vi "stable test.vi"() -> ()   [LabVIEW 2016]
uses:
  <vilib>/DAQmx/read.llb/DAQmx Read (Analog Wfm 1Chan NSamp).vi
  <vilib>/DAQmx/miscellaneous.llb/DAQmx Fill In Error Info.vi
  <resource>/objmgr/daqmx.rc
panel:
  out "data 2":waveform(dbl)
  out "Waveform Graph":waveform(dbl)(graph)
  out "data":dbl[](array[numeric]) format="%0.2f"
  out "error out":errorcluster
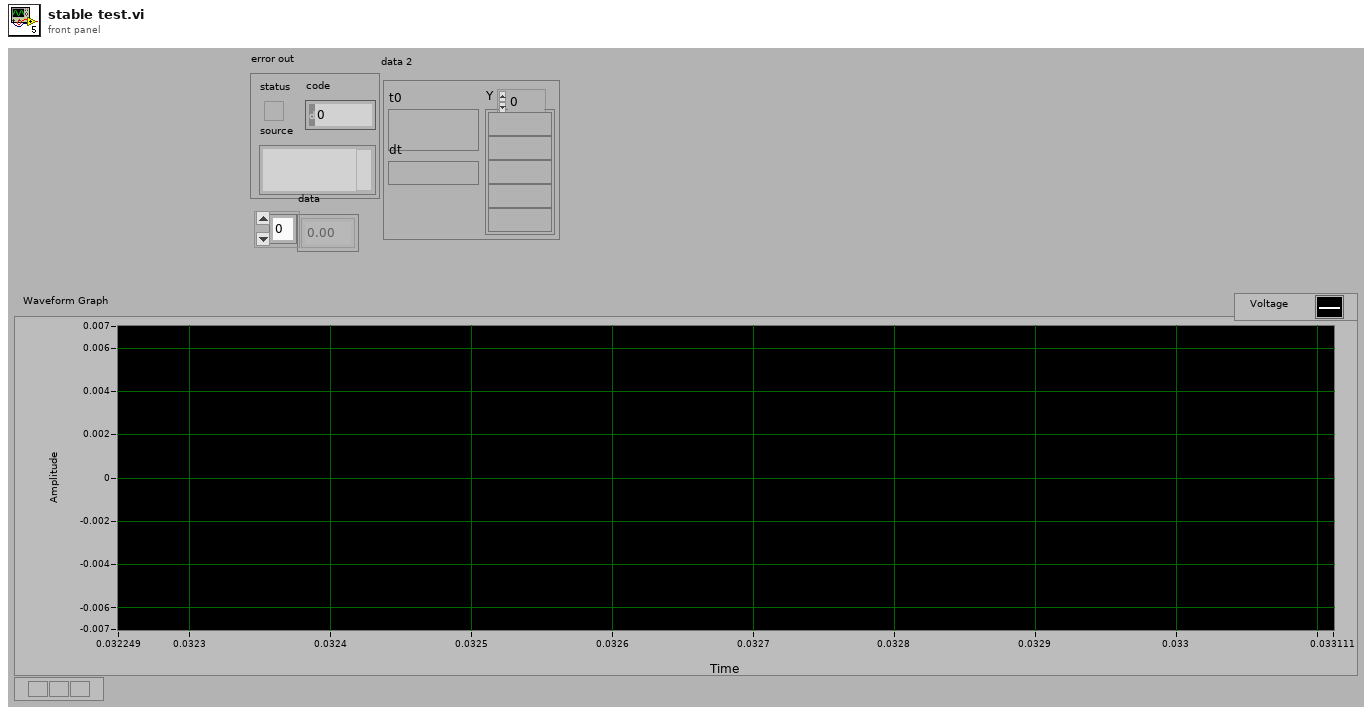
[diagram p1: front panel]
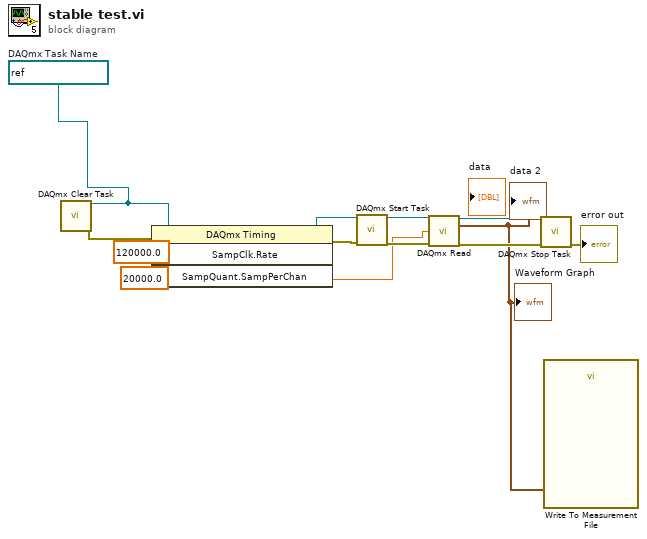
[diagram p0: block diagram]
diagram:
  w2 = 20000.0 ("SampClk.Rate")
  w10 = refnum<k21> "testcurrent"  # DAQmx Task Name
  n1 = call <vilib>:"DAQmx Clear Task.vi"("task in"=w10) -> ("error out"=w12:errorcluster)  [unwired: 14 in]
  n2 = property class="DAQmx Timing"(reference=w10, error in=w12, "SampClk.Rate"=120000.0, "SampQuant.SampPerChan"=w2) -> (reference out=w9:refnum<k21>, error out=w8:errorcluster)
  n3 = call <vilib>:"DAQmx Start Task.vi"("task/channels in"=w9, "error in"=w8) -> ("task out"=w6:refnum<k21>, "error out"=w7:errorcluster)  [unwired: 12 in]
  n4 = call-poly <vilib>:"DAQmx Read.vi"("task/channels in"=w6, "number of samples per channel"=w2, "error in"=w7) -> ("task out"=w4:refnum<k21>, "data"=w1:waveform(dbl), "error out"=w5:errorcluster)  [unwired: 10 in]
  "Waveform Graph" <- w1
  "data 2" <- w1
  n5 = call <vilib>:"DAQmx Stop Task.vi"("task/channels in"=w4, "error in"=w5) -> ("error out"=→"error out":errorcluster)  [unwired: 12 in, 1 out]
  n6 = call "Write To Measurement File"("Signals"=w1) -> ()  [unwired: 16 in, 3 out]
